vi "Export State.vi"(0 "SystemLink connection in":T1, 5 "state name":string, 11 "error in (no error)":errorcluster) -> (4 "SystemLink connection out":T1, 6 "state name out":string, 8 "raw state text":string, 15 "error out":errorcluster)   [LabVIEW 2017, in "SystemLink_States_API.lvlib"]
doc: "Exports the raw state text of the specified state.\n\nNote: To create a state file, write the raw state text to a text file and save the text file with a .sls file extension."
uses:
  SystemLink_States_API.lvlib
  _support/systemlink repo.ctl
  <vilib>/httpClient/ClientHandle.ctl
  <vilib>/httpClient/POSTBuffer.vi
  <vilib>/httpClient/LabVIEWHTTPClient.lvlib
panel:
  out "headers":string
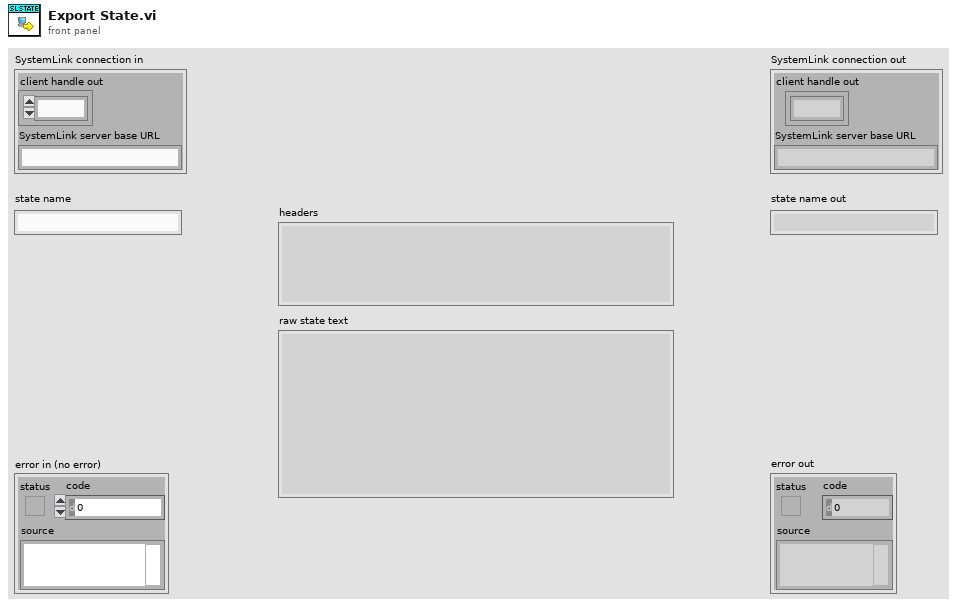
[diagram p1: front panel]
types:
  T1 = typedef "SystemLink_States_API.lvlib/systemlink repo.ctl" = cluster{"client handle out":T2, "SystemLink server base URL":string}
  T2 = typedef "LabVIEWHTTPClient.lvlib/ClientHandle.ctl" = refnum<k1>
  T3 = cluster{"inline":bool, "state":cluster{"stateID":string, "stateVersion":string}}
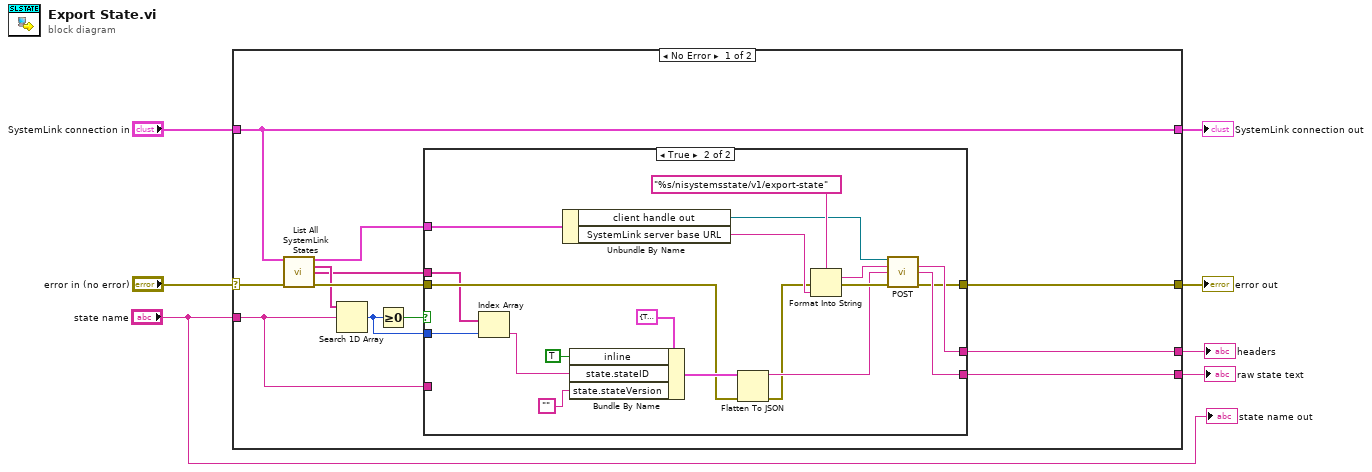
[diagram p0: block diagram]
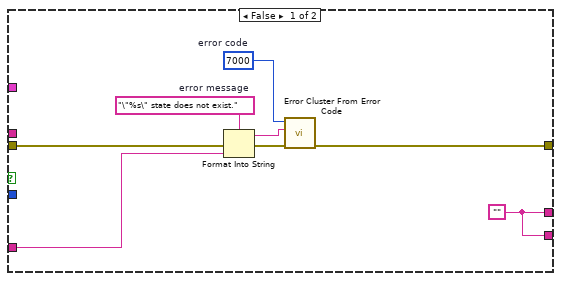
[diagram p2: hidden frame]
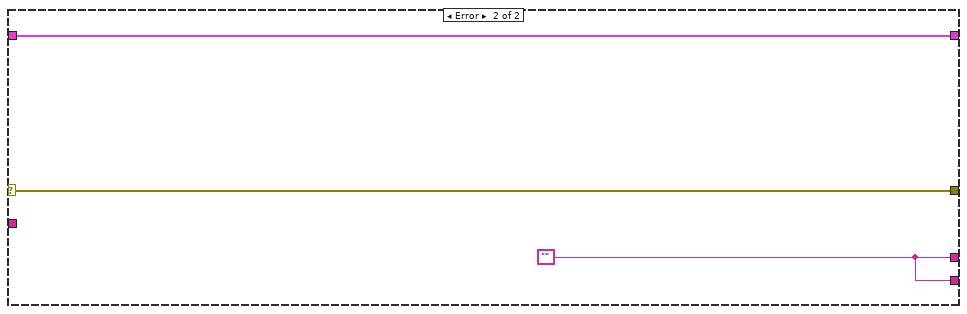
[diagram p3: hidden frame]
diagram:
  n1 = case shown="No Error" "error in (no error)" {
    selector: "error in (no error)" -> [w16 w49]
    tunnel: "SystemLink connection in" -> [w14 w48]
    tunnel: [w17 w49] -> w5
    tunnel: [w19 w47] -> w4
    tunnel: [w18 w47] -> w3
    tunnel: [w14 w48] -> w2
    tunnel: "state name" -> [w8 _]
    frame No Error {
      n2 = call "List All SystemLink States.vi"("SystemLink connection in"=w14, "error in (no error)"=w16) -> ("SystemLink connection out"=w13:T1, "SystemLink State Names"=w12:string[], "SystemLink State IDs"=w10:string[], "error out"=w15:errorcluster)  [unwired: 10 in]
      n3 = Search 1D Array(1D array=w12, element=w8) -> (index of element=w9:i32)  [unwired: 1 in]
      n4 = Greater Or Equal To 0?(x=w9) -> (x >= 0?=w11:bool)
      n5 = case shown="True" w11 {
        tunnel: [w20 w46] -> w19
        tunnel: [w20 w45] -> w18
        tunnel: [w27 w37] -> w17
        tunnel: w15 -> [w22 w32]
        tunnel: w13 -> [_ w31]
        tunnel: w10 -> [_ w30]
        tunnel: w9 -> [_ w29]
        tunnel: w8 -> [w24 _]
        frame False {
          w20 = ""
          w25 = "\"%s\" state does not exist."  # error message
          w26 = 7000  # error code
          n6 = Format Into String(format string=w25, error in=w22, w24) -> (resulting string=w23:string, error out=w21:errorcluster)  [unwired: 1 in]
          n7 = call <vilib>:"Error Cluster From Error Code.vi"("error in (no error)"=w21, "error message (\"\")"=w23, "error code (0)"=w26) -> ("error out"=w27:errorcluster)  [unwired: 6 in]
        }
        frame True {
          n8 = Index Array(array=w30, index=w29) -> (element=w28:string)
          n9 = Unbundle By Name(w31) -> ("client handle out"=w42:T2, "SystemLink server base URL"=w40:string)
          n10 = Bundle By Name(cluster=T3 {"inline"=TRUE, "state"={"stateID"="", "stateVersion"=""}}, "inline"=TRUE, "state.stateID"=w28, "state.stateVersion"="") -> (w35:T3)
          n11 = Flatten To JSON(anything=w35, error in (no error)=w32) -> (JSON string=w39:string, 11:w38:errorcluster)  [unwired: 1 in]
          n12 = Format Into String(format string="%s/nisystemsstate/v1/export-state", error in=w38, w40) -> (resulting string=w43:string, error out=w41:errorcluster)  [unwired: 1 in]
          n13 = call-poly <vilib>:"POST.vi"("client handle"=w42, "url"=w43, "buffer"=w39, "error in (no error)"=w41) -> ("headers"=w45:string, "body"=w46:string, "error out"=w37:errorcluster)  [unwired: 8 in, 1 out]
        }
      }
    }
    frame Error {
      w47 = "" ("headers")
    }
  }
  "error out" <- w5
  "SystemLink connection out" <- w2
  "headers" <- w3
  "raw state text" <- w4
  "state name out" <- "state name"
